vi "test.vi"() -> ()   [LabVIEW 2019]
panel:
  out "sin(x)":dbl
  out "concatenated string":string
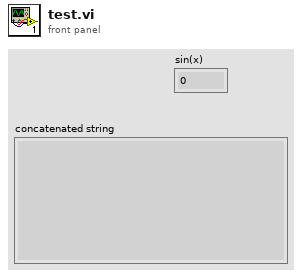
[diagram p1: front panel]
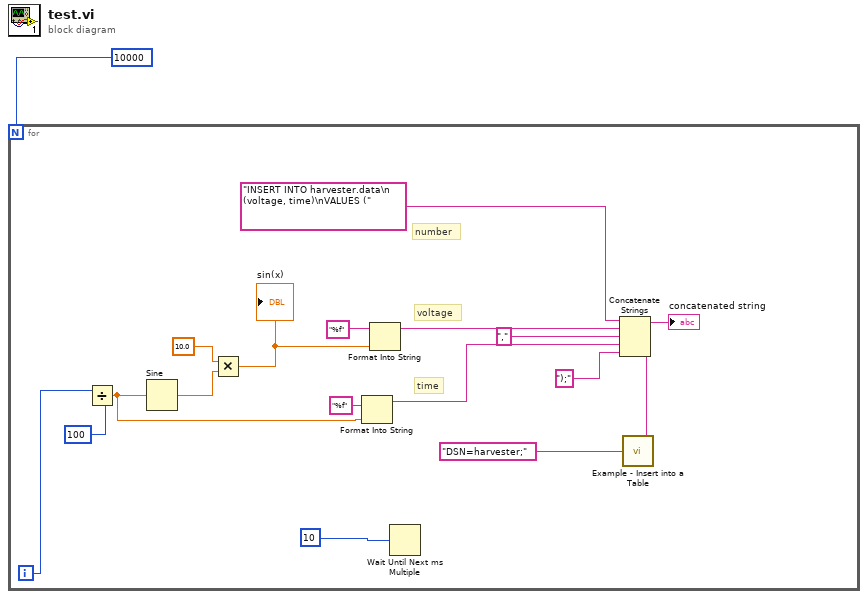
[diagram p0: block diagram]
diagram:
  n1 = for {
    N: 10000 -> [_]
    i -> [w12]
    # "time"
    # "voltage"
    # "number"
    n2 = Divide(x=w12, y=100) -> (x/y=w10:dbl)
    n3 = Sine(x=w10) -> (sin(x)=w4:dbl)
    n4 = Multiply(x=10.0, y=w4) -> (x*y=w2:dbl)
    "sin(x)" <- w2
    n5 = Format Into String(format string="%f", w10) -> (resulting string=w7:string)  [unwired: 2 in, 1 out]
    n6 = Format Into String(format string="%f", w2) -> (resulting string=w9:string)  [unwired: 2 in, 1 out]
    n7 = Wait Until Next ms Multiple(millisecond multiple=u32 10 ("millisecond timer value")) -> ()  [unwired: 1 out]
    n8 = Concatenate Strings("INSERT INTO harvester.data\n (voltage, time)\nVALUES (", w9, "," ("string"), w7, ");" ("string")) -> (w13:string)
    "concatenated string" <- w13
    n9 = call "Example - Insert into a Table.vi"("Command Text"=w13, "ConnectionString"="DSN=harvester;" ("Command Text")) -> ()
  }
